vi "ERR HANDLER - Error Status FGV.vi"(7 "Method":enum16{"READ", "WRITE"}(ring), 9 "Abort Program (W)":enum16{"Not Yet", "ABORT"}(ring), 10 "Last Error (W)":errorcluster, 11 "Error Count (W)":i32) -> (1 "Abort Program (R)":enum16{"Not Yet", "ABORT"}(ring), 2 "Last Error (R)":errorcluster, 3 "Error Count (R)":i32)   [LabVIEW 2013]
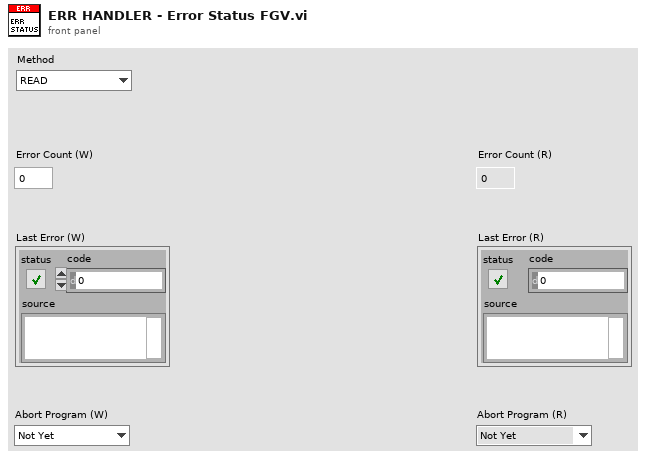
[diagram p1: front panel]
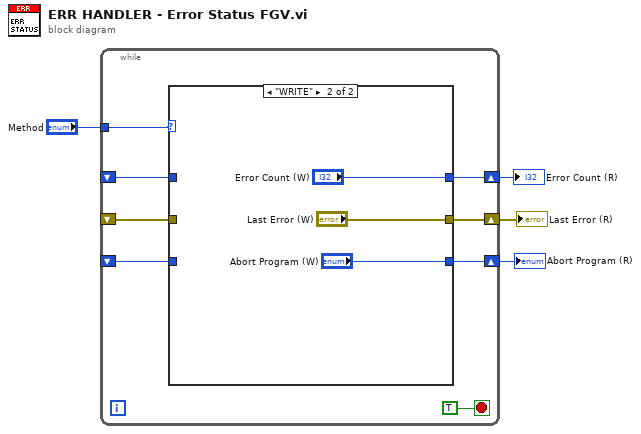
[diagram p0: block diagram]
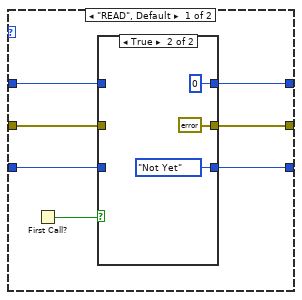
[diagram p2: hidden frame]
diagram:
  n1 = while {
    shift-right: [w10] -> w1
    shift-left: _ -> [w8]
    tunnel: "Method" -> [w11]
    shift-right: [w9] -> w3
    shift-left: _ -> [w7]
    shift-right: [w6] -> w2
    shift-left: _ -> [w5]
    stop <- TRUE stop-if-true
    n2 = case shown="\"WRITE\"" w11 {
      tunnel: [w15 "Error Count (W)"] -> w10
      tunnel: [w14 "Last Error (W)"] -> w9
      tunnel: w8 -> [w18 _]
      tunnel: w7 -> [w17 _]
      tunnel: [w13 "Abort Program (W)"] -> w6
      tunnel: w5 -> [w16 _]
      frame "READ", Default {
        n3 = First Call?() -> (First Call?: T/F=w19:bool)
        n4 = case shown="True" w19 {
          tunnel: w18 -> [w22 _]
          tunnel: w17 -> [w21 _]
          tunnel: w16 -> [w20 _]
          tunnel: [w22 0 ("Error Count (W)")] -> w15
          tunnel: [w21 errorcluster {"status"=FALSE, "code"=0, "source"=""} ("Last Error (W)")] -> w14
          tunnel: [w20 enum16{"Not Yet", "ABORT"}."Not Yet" ("Abort Program (W)")] -> w13
          frame False {
          }
          frame True {
          }
        }
      }
      frame "WRITE" {
      }
    }
  }
  "Last Error (R)" <- w3
  "Abort Program (R)" <- w2
  "Error Count (R)" <- w1
